vi "LAC Cmd_Excution.vi"(7 "timeout(ms)":u32=500, 8 "error in":errorcluster, 10 "Cmd_exec":T1=100 items=["Stop meas."=100, "Start meas."=99, "Auto-adj. LD output"=105, "Zero reset"=106, "Zero set"=107, "OFFSETTILT judge 1"=108, "OFFSETTILT judge 2"=109], 11 "VISA name in":refnum<visa-resource-name>) -> (0 "error out":errorcluster, 1 "read buffer":string, 3 "VISA name out":refnum<visa-resource-name>)   [LabVIEW 2018]
uses:
  TypeDef/H410 Cmd_exec TypeDef.ctl
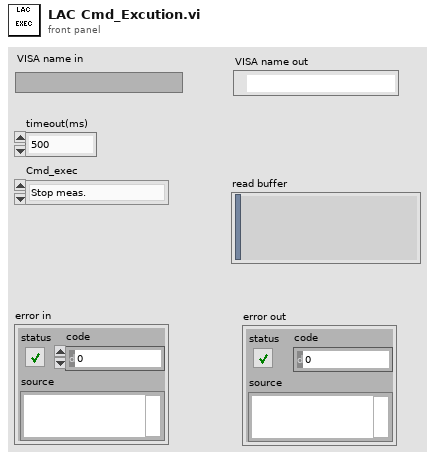
[diagram p1: front panel]
types:
  T1 = typedef "H410 Cmd_exec TypeDef.ctl" = u16
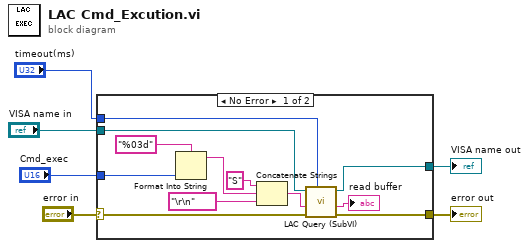
[diagram p0: block diagram]
diagram:
  n1 = case shown="No Error" "error in" {
    selector: "error in" -> [w13 w20]
    tunnel: "VISA name in" -> [w15 w19]
    tunnel: [w18 w19] -> w5
    tunnel: [w16 w20] -> w4
    tunnel: "timeout(ms)" -> [w14 _]
    tunnel: "Cmd_exec" -> [w9 _]
    frame No Error {
      n2 = Format Into String(format string="%03d", w9) -> (resulting string=w7:string)  [unwired: 2 in, 1 out]
      n3 = Concatenate Strings("S" ("string"), w7, "\r\n" ("write buffer")) -> (w11:string)
      n4 = call "LAC Query (SubVI).vi"("timeout(ms)"=w14, "error in"=w13, "Command"=w11, "VISA name in"=w15) -> ("error out"=w16:errorcluster, "read buffer"=→"read buffer":string, "VISA name out"=w18:refnum<visa-resource-name>)  [unwired: 5 in]
    }
    frame Error {
    }
  }
  "VISA name out" <- w5
  "error out" <- w4
